vi "Write u32FlagImpairmentArray.vi"(8 "error in (no error)":errorcluster, 10 "u32FlagImpairmentArray":T1, 11 "OutputToFileBasePlugin in":refnum<class "OutputToFileBasePlugin.lvclass">) -> (0 "error out":errorcluster, 3 "OutputToFileBasePlugin out":refnum<class "OutputToFileBasePlugin.lvclass">)   [LabVIEW 2017, in "OutputToFilePlugins.lvlib" / "OutputToFileBasePlugin.lvclass"]
uses:
  OutputToFileBasePlugin.lvclass
  FlagImpairPlugins/FlagImpairPluginBase_class/TypeDefs/FlagImpairmentArray.ctl
  OutputToFileBasePlugin.lvclass/OutputToFileBasePlugin.ctl
  FlagImpairPlugins/FlagImpairPluginBase_class/FlagImpairPluginBase.lvclass
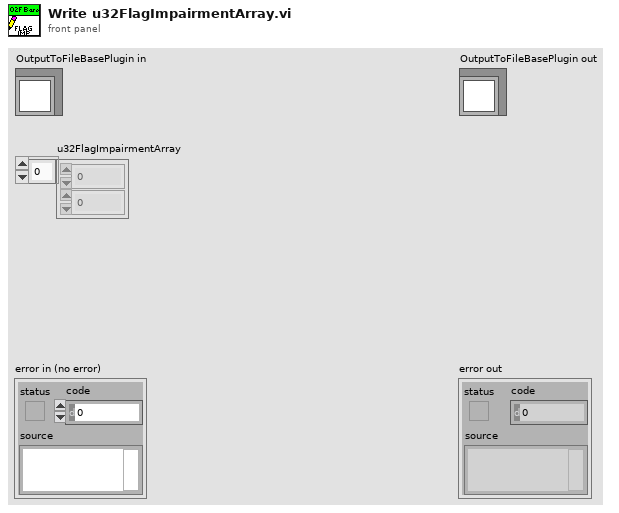
[diagram p1: front panel]
types:
  T1 = typedef "FlagImpairPlugins.lvlib/FlagImpairPluginBase.lvclass/FlagImpairmentArray.ctl" = u32[]
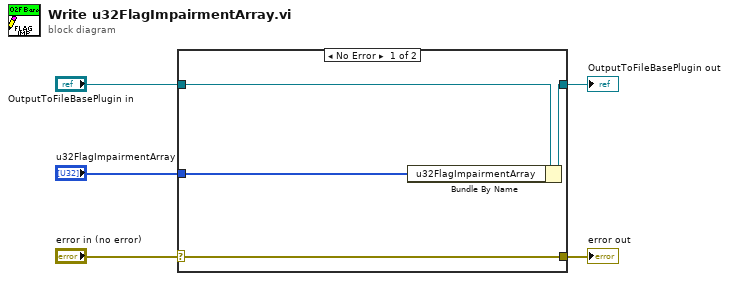
[diagram p0: block diagram]
diagram:
  n1 = case shown="No Error" "error in (no error)" {
    selector: "error in (no error)" -> [w9 w10]
    tunnel: [w9 w10] -> w4
    tunnel: [w7 w11] -> w2
    tunnel: "OutputToFileBasePlugin in" -> [w8 w11]
    tunnel: "u32FlagImpairmentArray" -> [w6 _]
    frame No Error {
      n2 = Bundle By Name(cluster=w8, "u32FlagImpairmentArray"=w6) -> (w7:refnum<class "OutputToFileBasePlugin.lvclass">)
    }
    frame Error {
    }
  }
  "error out" <- w4
  "OutputToFileBasePlugin out" <- w2
